vi "GetHold.vi"(6 "Legacy (f)?":bool, 8 "error in (no error)":errorcluster) -> (0 "error out":errorcluster, 2 "Hold":bool)   [LabVIEW 2011]
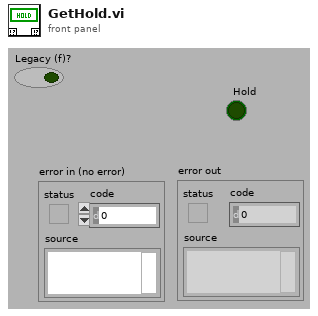
[diagram p1: front panel]
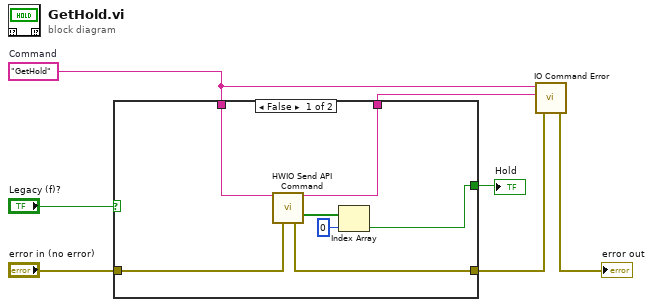
[diagram p0: block diagram]
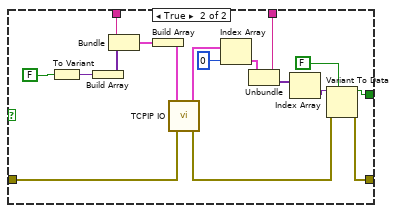
[diagram p2: hidden frame]
diagram:
  w5 = "GetHold"  # Command
  n1 = case shown="False" "Legacy (f)?" {
    tunnel: [w8 w27] -> w7
    tunnel: w5 -> [w14 w24]
    tunnel: [w13 w23] -> w4
    tunnel: "error in (no error)" -> [w12 w15]
    tunnel: [w11 w16] -> w1
    frame False {
      n2 = call "HWIO Send API Command.vi"("Action"=w14, "error in (no error)"=w12) -> ("Action out"=w13:string, "Boolean out"=w10:bool[], "error out"=w11:errorcluster)  [unwired: 6 in, 5 out]
      n3 = Index Array(array=w10, index=0) -> (element=w8:bool)
    }
    frame True {
      n4 = To Variant(anything=FALSE) -> (Variant=w31:variant)
      n5 = Build Array(w31) -> (w30:variant[])
      n6 = Bundle("Command"=w24, w30) -> (w29:cluster{"Command":string, variant[]})  [unwired: 1 out]
      n7 = Build Array(w29) -> (w26:cluster{"Command":string, variant[]}[])
      n8 = call "TCPIP IO.vi"("error in (no error)"=w15, "Commands"=w26) -> ("error out"=w25:errorcluster, "Responses"=w22:cluster{string, variant[]}[])  [unwired: 1 in, 3 out]
      n9 = Index Array(array=w22, index=0) -> (element=w21:cluster{string, variant[]})
      n10 = Unbundle(w21) -> (w23:string, w20:variant[])
      n11 = Index Array(array=w20) -> (element=w19:variant)  [unwired: 1 in]
      n12 = Variant To Data(error in=w25, type=FALSE, Variant=w19) -> (data=w27:bool, error out=w16:errorcluster)
    }
  }
  "Hold" <- w7
  n13 = call "IO Command Error.vi"("error in (no error)"=w1, "Command Returned (\"\")"=w4, "Command Sent (\"\")"=w5) -> ("error out"=→"error out":errorcluster)  [unwired: 4 out]
